vi "ex2_analog.vi"() -> ()   [LabVIEW 2018]
panel:
  in  "Slide":dbl(slide) scale=0.0..10.0
  out "Meter":dbl(knob) scale=0.0..10.0
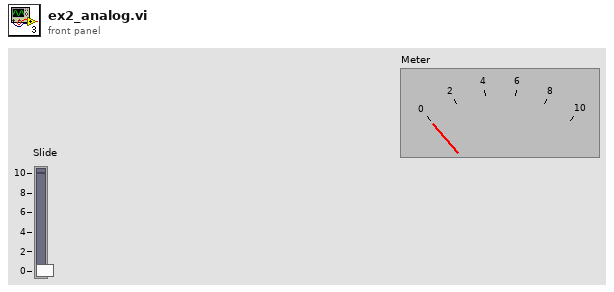
[diagram p1: front panel]
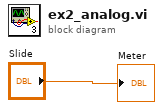
[diagram p0: block diagram]
diagram:
  "Meter" <- "Slide"
